vi "23384_Davis_Poku_Amankwa_Amankwa.DavisPoku.MNE1201.1.7_348252_2034381276.vi"() -> ()   [LabVIEW 2018]
panel:
  out "Outcome":string
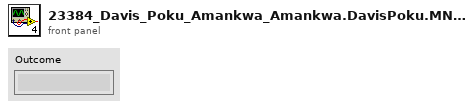
[diagram p1: front panel]
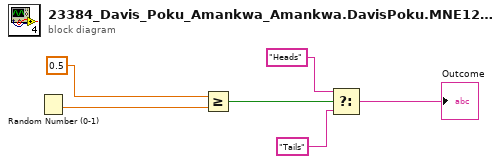
[diagram p0: block diagram]
diagram:
  n1 = Random Number (0-1)() -> (number: 0 to 1=w6:dbl)
  n2 = Greater Or Equal?(x=0.5, y=w6) -> (x >= y?=w4:bool)
  n3 = Select(t="Heads", s=w4, f="Tails") -> (s? t:f=→"Outcome":string)
